vi "DMM Acq Done.vi"(9 "Acquisition State":T1, 10 "Backlog":i32) -> (2 "Finished with Backlog?":bool, 3 "Sequence Acquision Finished?":bool)   [LabVIEW 2019, in "SupportVIs.lvlib"]
uses:
  SupportVIs.lvlib
  <instrlib>/niDMM/nidmm.llb/niDMM Acquisition State.ctl
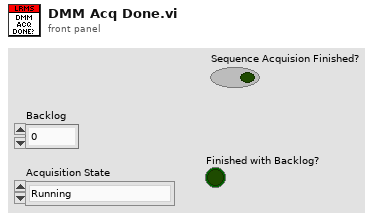
[diagram p1: front panel]
types:
  T1 = typedef "niDMM Acquisition State.ctl" = enum16{"Running", "Finished with Backlog", "Finished with no Backlog", "Paused", "No acquisition in progress"}
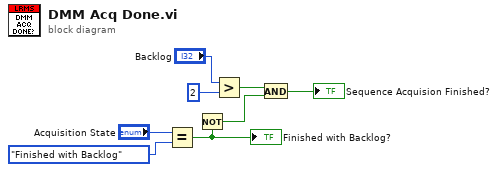
[diagram p0: block diagram]
diagram:
  n1 = Equal?(x="Acquisition State", y=niDMM_Acquisition_State."Finished with Backlog") -> (x = y?=w2:bool)
  "Finished with Backlog?" <- w2
  n2 = Not(x=w2) -> (.not. x?=w3:bool)
  n3 = Greater?(x="Backlog", y=2) -> (0:w7:bool)
  n4 = And(x=w7, y=w3) -> (x .and. y?=→"Sequence Acquision Finished?":bool)
